vi "Measurement.vi"() -> ()   [LabVIEW 2013]
panel:
  out "Player Array from reference":dbl[][](array[numeric])
  out "Puck Array From reference":dbl[][](array[numeric])
  in  "Calibrate":bool
  out "Binary":T1(plugin-control)
  out "Histogram":T2(graph)
  out "Image in":T1(plugin-control)
  in  "Stop":bool
  in  "Capture image":bool
  out "Calibrated":T1(plugin-control)
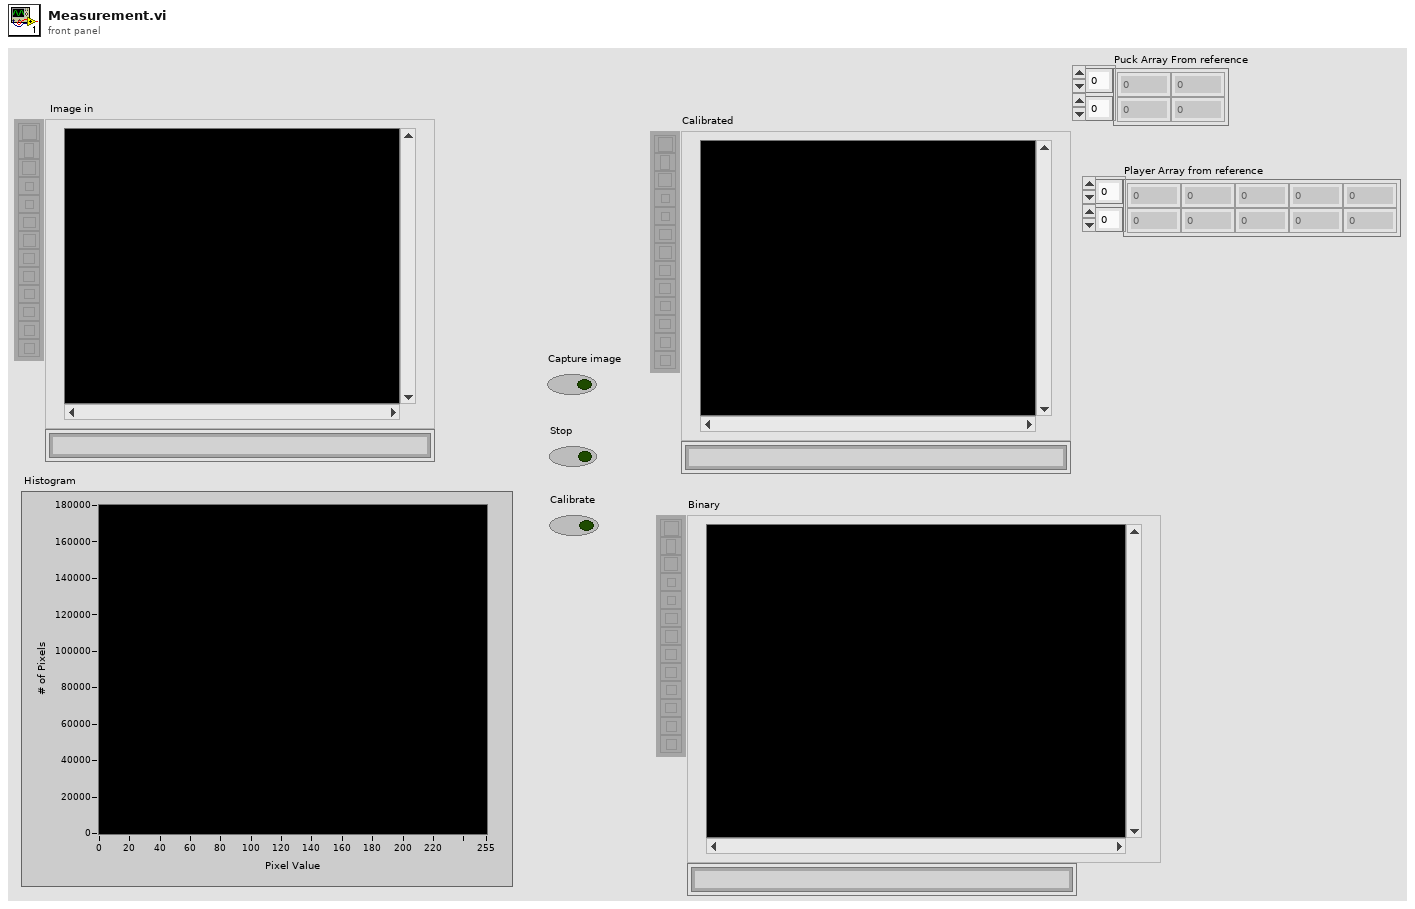
[diagram p1: front panel]
types:
  T1 = typedef "IMAQ Image.ctl" = refnum<image>
  T2 = cluster{"Starting Value":sgl, "Incremental Value":sgl, "Histogram":u32[]}
  T3 = cluster{"Point1 (Pixels)":cluster{"X":sgl, "Y":sgl}, "Point2 (Pixels)":cluster{"X":sgl, "Y":sgl}, "Point1 (Real-World)":cluster{"X":sgl, "Y":sgl}, "Point2 (Real-World)":cluster{"X":sgl, "Y":sgl}, "Angle (Pixel)":dbl, "Angle (Real-World)":dbl, "Score":dbl, "Straightness":dbl, "Average SNR (db)":dbl, "Calibration Valid":bool}
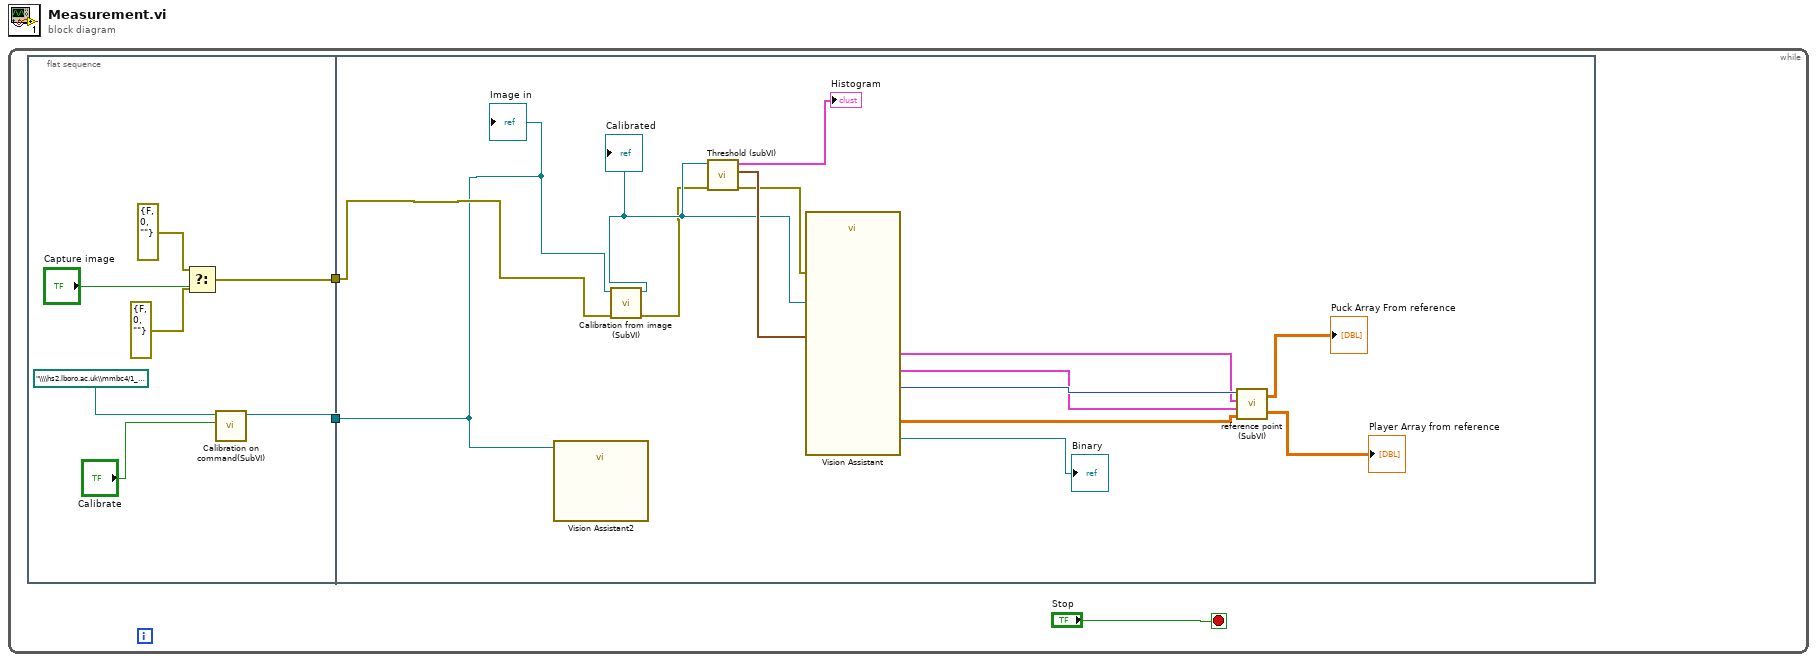
[diagram p0: block diagram]
diagram:
  n1 = while {
    stop <- "Stop" stop-if-true
    n2 = flat-sequence {
      tunnel: [w7] -> w2
      tunnel: [w5] -> w1
      tunnel: w2 -> [w18]
      tunnel: w1 -> [w11]
      frame #0 {
        n3 = Select(t=errorcluster {"status"=FALSE, "code"=0, "source"=""} ("error in"), s="Capture image", f=errorcluster {"status"=FALSE, "code"=0, "source"=""} ("error in")) -> (s? t:f=w7:errorcluster)
        n4 = call "Calibration on command(SubVI).vi"("Calibrate"="Calibrate", "File Path (Image Calibration 1)"=path "\\\\hs2.lboro.ac.uk\\mmbc4/1_Univesity Work/Mechatronics/Machine Vision/2.0_Harry_kane/Auto_calibration.png") -> ("Refnum out"=w5:T1)  [unwired: 8 in, 1 out]
      }
      frame #1 {
        n5 = call "Vision Assistant2"("Image In"=w11) -> ()  [unwired: 25 in, 2 out]
        n6 = call "Calibration from image (SubVI).vi"("error in (no error)"=w18, "Refnum in"=w11) -> ("error out"=w16:errorcluster, "Refnum out"=w17:T1)  [unwired: 8 in]
        "Calibrated" <- w17
        n7 = call "Threshold (subVI).vi"("error in (no error)"=w16, "Image  in"=w17) -> ("error out"=w15:errorcluster, "Cluster"=w24:cluster{sgl, "element":sgl}, "Histogram"=→"Histogram":T2)  [unwired: 7 in]
        n8 = call "Vision Assistant"("Image In"=w17, "Range (Threshold 1)"=w24, "error in"=w15) -> ("Image Out"=→"Binary":T1, "Particle Measurements (Real-World) (Particle Analysis 1)"=w14:dbl[][], "Straight Edge (Find Straight Edge 1)"=w20:T3, "Straight Edge (Find Straight Edge 2)"=w19:T3, "Nb Circles (Circle Detection 1)"=w21:i32)  [unwired: 18 in, 2 out]
        n9 = call "reference point (SubVI).vi"("Nb Circles (Circle Detection 1)"=w21, "Straight Edge (Find Straight Edge 1)"=w20, "Straight Edge (Find Straight Edge 2)"=w19, "Particle Measurements (Real-World) (Particle Analysis 1)"=w14) -> ("Puck X, Y co-ordinates"=→"Puck Array From reference":dbl[][], "Player X, Y co-ordinates"=→"Player Array from reference":dbl[][])  [unwired: 1 in]
        "Image in" <- w11
      }
    }
  }
